vi "Serial_GetComs&PortDescriptions.vi"(8 "error in (no error)":errorcluster) -> (0 "error out":errorcluster, 2 "WinsDescriptions":string[](array[string]), 3 "COMs":refnum<visa-resource-name>[](array[refnum]))   [LabVIEW 2020, in "NOYITO 10 Channel ADC Module Driver.lvlib"]
uses:
  <vilib>/Instr/_visa.llb/VISA Find Search Mode.ctl
  NOYITO 10 Channel ADC Module Driver.lvlib
panel:
  out "find list":string[](array[string])
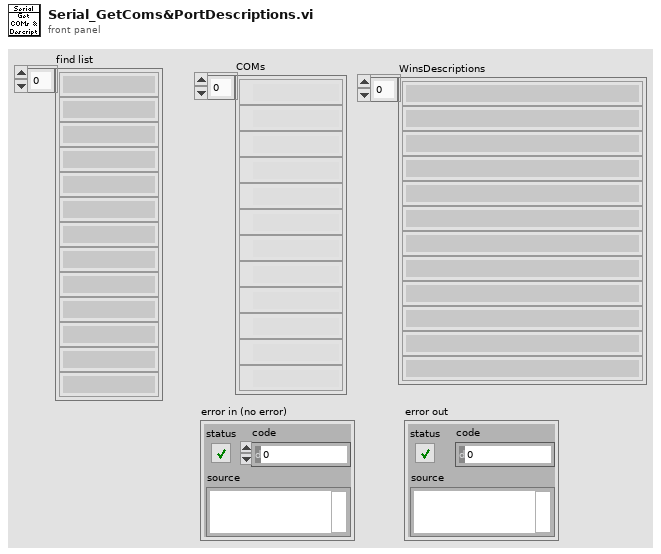
[diagram p1: front panel]
types:
  T1 = typedef "VISA Find Search Mode.ctl" = u32
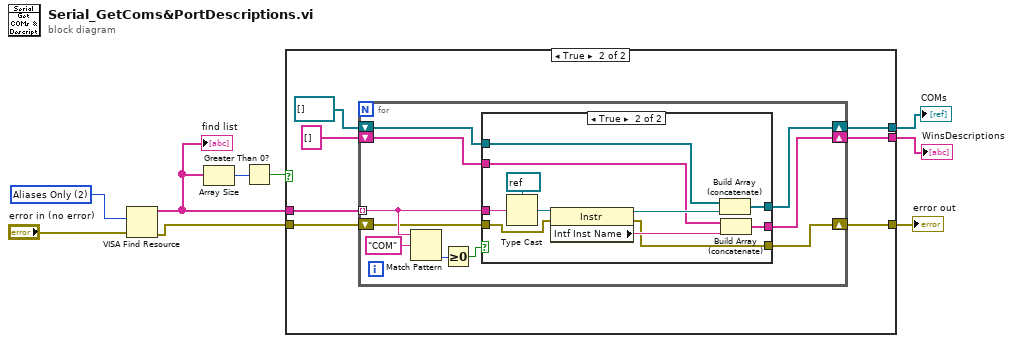
[diagram p0: block diagram]
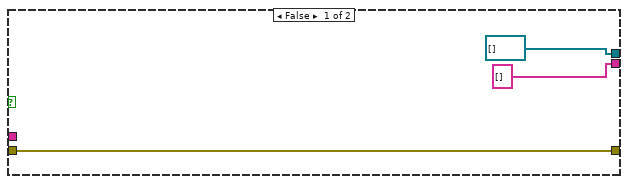
[diagram p2: hidden frame]
diagram:
  w9 = T1 2 items=["Canonical Names Only"=0, "Aliases Only"=2, "Include Matching Aliases"=3, "Include All Aliases"=4] ("Search Mode")
  n1 = VISA Find Resource(8:"error in (no error)", 10:w9) -> (0:w2:errorcluster, 3:w6:string[])  [unwired: 1 in, 1 out]
  "find list" <- w6
  n2 = Array Size(array=w6) -> (size(s)=w5:i32)
  n3 = Greater Than 0?(x=w5) -> (x > 0?=w4:bool)
  n4 = case shown="True" w4 {
    tunnel: [refnum<visa-resource-name>[] [] w19] -> w8
    tunnel: [string[] [] w18] -> w7
    tunnel: w6 -> [_ w17]
    tunnel: w2 -> [w10 w14]
    tunnel: [w10 w13] -> w1
    frame False {
    }
    frame True {
      n5 = for {
        tunnel: w17 -> [w29] mode=indexing
        shift-right: [w24] -> w19
        shift-left: refnum<visa-resource-name>[] [] -> [w25]
        shift-right: [w22] -> w18
        shift-left: string[] [] -> [w23]
        shift-right: [w20] -> w13
        shift-left: w14 -> [w21]
        n6 = Match Pattern(string=w29, regular expression="COM") -> (offset past match=w27:i32)  [unwired: 1 in, 3 out]
        n7 = Greater Or Equal To 0?(x=w27) -> (x >= 0?=w26:bool)
        n8 = case shown="True" w26 {
          tunnel: w29 -> [_ w42]
          tunnel: w23 -> [w32 w36]
          tunnel: w25 -> [w31 w35]
          tunnel: [w31 w39] -> w24
          tunnel: [w32 w37] -> w22
          tunnel: w21 -> [w30 w34]
          tunnel: [w30 w33] -> w20
          frame False {
          }
          frame True {
            n9 = Type Cast(type=refnum<visa-resource-name> refnum ("VISA resource name"), x=w42) -> (*(type *) &x=w41:refnum<visa-resource-name>)
            n10 = property class="Instr"(reference=w41, error in=w34) -> (reference out=w40:refnum<visa-resource-name>, error out=w33:errorcluster, "Intf Inst Name"=w38:string)
            n11 = Build Array (concatenate)(w35, w40) -> (w39:refnum<visa-resource-name>[])
            n12 = Build Array (concatenate)(w36, w38) -> (w37:string[])
          }
        }
      }
    }
  }
  "COMs" <- w8
  "WinsDescriptions" <- w7
  "error out" <- w1
